vi "LVProjectShortcut_WriteProperties.vi"(6 "hasPath":bool=TRUE, 8 "error in":errorcluster, 9 "filePath":path, 10 "shortcutName":string, 11 "Wizard":T1) -> (0 "error out":errorcluster)   [LabVIEW 2017, in "LVProject Shortcut.lvlib"]
uses:
  <resource>/Framework/Providers/API/ItemRef.ctl
  <resource>/Framework/Providers/API/mxLvSetBooleanProperty.vi
  <resource>/Framework/Providers/API/mxLvSetStringProperty.vi
  LVProject Shortcut.lvlib
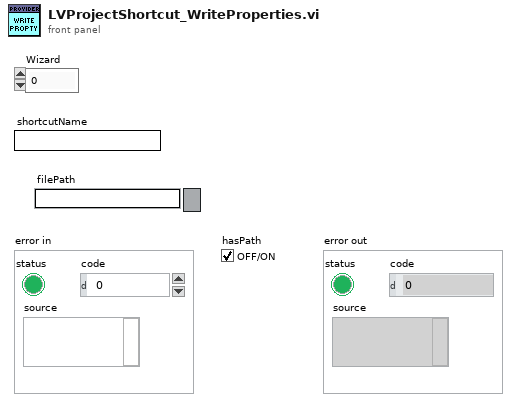
[diagram p1: front panel]
types:
  T1 = typedef "ItemRef.ctl" = u64
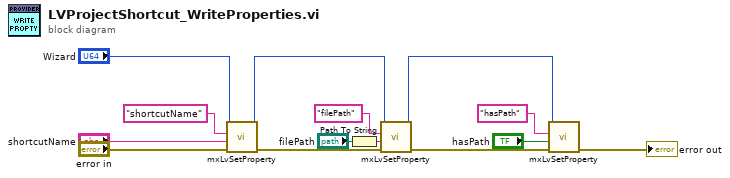
[diagram p0: block diagram]
diagram:
  n1 = call-poly <resource>:"mxLvSetProperty.vi"("error in"="error in", "Value (\"\")"="shortcutName", "Tag"="shortcutName", "Item"="Wizard") -> ("error out"=w10:errorcluster, "Item"=w7:T1)  [unwired: 6 in]
  n2 = Path To String(path="filePath") -> (string=w1:string)
  n3 = call-poly <resource>:"mxLvSetProperty.vi"("error in"=w10, "Value (\"\")"=w1, "Tag"="filePath", "Item"=w7) -> ("error out"=w3:errorcluster, "Item"=w2:T1)  [unwired: 6 in]
  n4 = call-poly <resource>:"mxLvSetProperty.vi"("error in"=w3, "Value (F)"="hasPath", "Tag"="hasPath", "Item"=w2) -> ("error out"=→"error out":errorcluster)  [unwired: 6 in, 1 out]
